vi "niFpgaSupportedCompilationToolVersions.vi"() -> ()   [LabVIEW 2020]
uses:
  <vilib>/rvi/ClientSDK/Core/CompilationInfo/niFpgaCompilationToolVersion_data.ctl
  <vilib>/rvi/ClientSDK/Core/CompilationInfo/niFpgaCompilationToolVersion_compiler.ctl
  <vilib>/rvi/ClientSDK/Core/CompilationInfo/niFpgaCompilationToolVersion_bits.ctl
panel:
  in  "Default 64-bit Vivado":T1={"Compiler"=enum."Xilinx Vivado", "Bits"=enum."64bit", "Major Version"=2019, "Minor Version"=1}
  in  "Default 32-bit Vivado":T1={"Compiler"=enum."Xilinx Vivado", "Bits"=enum."32bit", "Major Version"=2015, "Minor Version"=4}
  in  "Default 64-bit ISE":T1={"Compiler"=enum."Xilinx ISE", "Bits"=enum."64bit", "Major Version"=14, "Minor Version"=7}
  in  "Default 32-bit ISE":T1={"Compiler"=enum."Xilinx ISE", "Bits"=enum."32bit", "Major Version"=14, "Minor Version"=7}
  in  "Legacy ISE for Virtex-2":T1={"Compiler"=enum."Xilinx ISE", "Bits"=enum."32bit", "Major Version"=10, "Minor Version"=1}
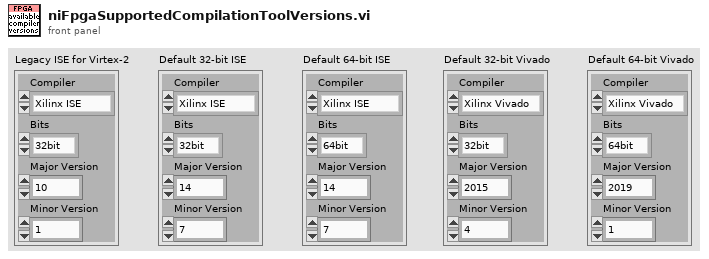
[diagram p1: front panel]
types:
  T1 = typedef "niFpgaCompilationToolVersion_data.ctl" = cluster{"Compiler":T2, "Bits":T3, "Major Version":i32, "Minor Version":i32}
  T2 = typedef "niFpgaCompilationToolVersion_compiler.ctl" = enum16{"Xilinx ISE", "Xilinx Vivado"}
  T3 = typedef "niFpgaCompilationToolVersion_bits.ctl" = enum16{"32bit", "64bit"}
diagram:
